vi "ex5-6.vi"   [LabVIEW 2014]
uses:
  <vilib>/NXT/Subs/MotorOutput.ctl
  <vilib>/NXT/Block Support/NXT_ButtonSelector.ctl
  <vilib>/NXT/Dual Mode Library/Motors/MotorOn.vi
  <vilib>/NXT/Dual Mode Library/Waits/Wait_Num.vi
  <vilib>/NXT/Dual Mode Library/Motors/MotorBrake.vi
types:
  T1 = typedef "LVHSConnector.ctl" = refnum<class "BrickReference.lvclass">
  T2 = typedef "NXT_ButtonSelector.ctl" = u16
  T3 = typedef "MotorOutput.ctl" = u8
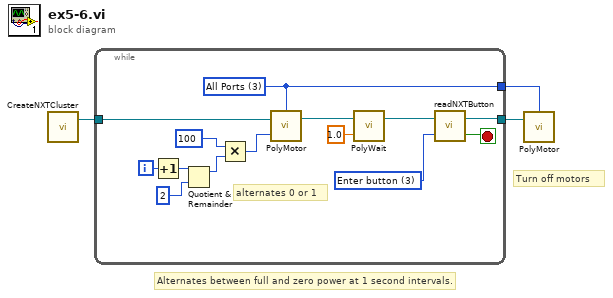
[diagram p0: block diagram]
diagram:
  # "Turn off motors"
  # "Alternates between full and zero power at 1 second intervals."
  n1 = call <vilib>:"CreateNXTCluster.vi"() -> ("NXT/EV3"=w3:T1)  [unwired: 4 in]
  n2 = while {
    tunnel: [w7] -> w2
    tunnel: w3 -> [w12]
    tunnel: [w6] -> w1
    i -> [w17]
    stop <- w5 stop-if-true
    w4 = T2 3 items=["Enter button"=3, "Left button"=2, "Right button"=1] ("Button (Enter button)")
    w7 = T3 3 items=["Port A", "Port B", "Port C", "All Ports"] ("Output Port")
    # "alternates 0 or 1"
    n3 = Increment(x=w17) -> (x+1=w13:i32)
    n4 = Quotient & Remainder(x=w13, y=2) -> (x-y*floor(x/y)=w15:i32)  [unwired: 1 out]
    n5 = Multiply(x=100, y=w15) -> (x*y=w9:i32)
    n6 = call-poly <vilib>:"PolyMotor.vi"("Power (75)"=w9, "NXT/EV3"=w12, "Output Port (All Ports)"=w7) -> ("NXT/EV3"=w11:T1)  [unwired: 1 out]
    n7 = call-poly <vilib>:"PolyWait.vi"("Time (1 sec)"=sgl 1.0 ("Time (sec)"), "NXT/EV3"=w11) -> ("NXT/EV3"=w10:T1)  [unwired: 2 out]
    n8 = call <vilib>:"readNXTButton.vi"("Button (Enter button)"=w4, "NXT/EV3"=w10) -> ("Yes/No"=w5:bool, "NXT/EV3"=w6:T1)  [unwired: 1 out]
  }
  n9 = call-poly <vilib>:"PolyMotor.vi"("NXT/EV3"=w1, "Port (All Ports)"=w2) -> ()  [unwired: 3 out]
